vi "LWXPS_SetTimeout.vi"(0 "XPS Reference IN":refnum<k24>, 2 "Sending Timeout":i32, 3 "Reading Timeout":i32, 5 "LabVIEW error IN":errorcluster) -> (6 "XPS Reference OUT":refnum<k24>, 7 "Returned error code":i32, 8 "LabVIEW error OUT":errorcluster)   [LabVIEW 2014]
uses:
  D:/XPSQ8_LabView_Library/Development/Source/Dll/Newport.XPS.CommandInterface.dll
  Dll/Newport.XPS.CommandInterface.dll
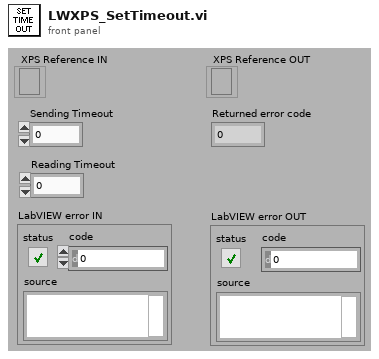
[diagram p1: front panel]
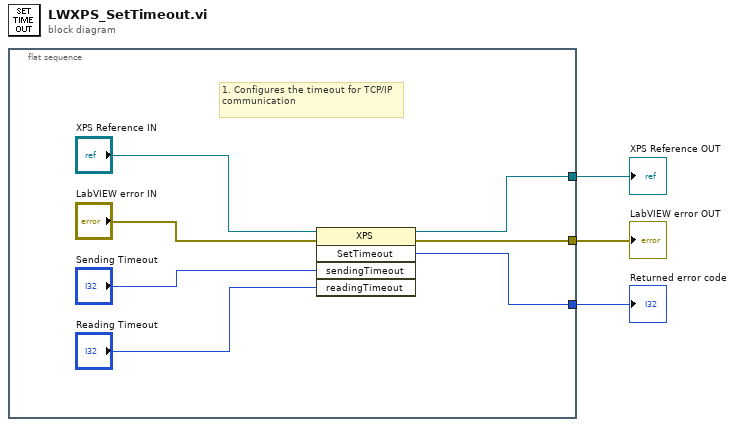
[diagram p0: block diagram]
diagram:
  n1 = flat-sequence {
    tunnel: [w8] -> w3
    tunnel: [w6] -> w2
    tunnel: [w9] -> w1
    frame #0 {
      # "1. Configures the timeout for TCP/IP communication"
      n2 = invoke class="XPS" method="SetTimeout"(reference="XPS Reference IN", error in="LabVIEW error IN", "sendingTimeout"="Sending Timeout", "readingTimeout"="Reading Timeout") -> (reference out=w8:refnum<k24>, error out=w6:errorcluster, "SetTimeout"=w9:i32)  [unwired: 1 in, 2 out]
    }
  }
  "XPS Reference OUT" <- w3
  "LabVIEW error OUT" <- w2
  "Returned error code" <- w1
